vi "S8300E_Button_Test_WIH.vi"() -> ()   [LabVIEW 2011]
panel:
  out "LOG2":string
  out "Debug View":string
  in  "NG STOP":bool
  out "Pass?":bool
  out "Log":string
  out "MSG List":string[](array[string])
  out "VISA resource name out":refnum<visa-resource-name>
  out "Cmd Line":cluster{string, string, "BIST Version":string}[](array[cluster])
  out "BEGIN TIME":u32
  out "進行狀況":string
  # "Error Code:Button\nError Code:UART"
  # "2015-6-2"
  # "ShutDown Button Check"
  # "COM9 :Baud-Rate:115200"
  # "Warning:Please follow the instruction to press the Shutdown Button"
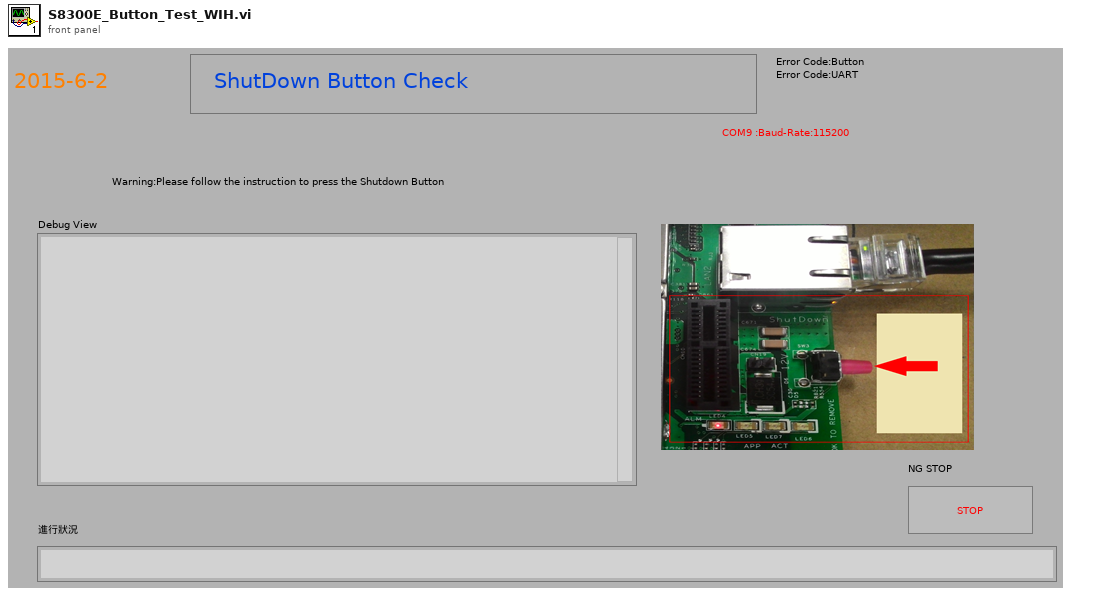
[diagram p1: front panel]
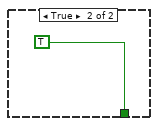
[diagram p4: hidden frame]
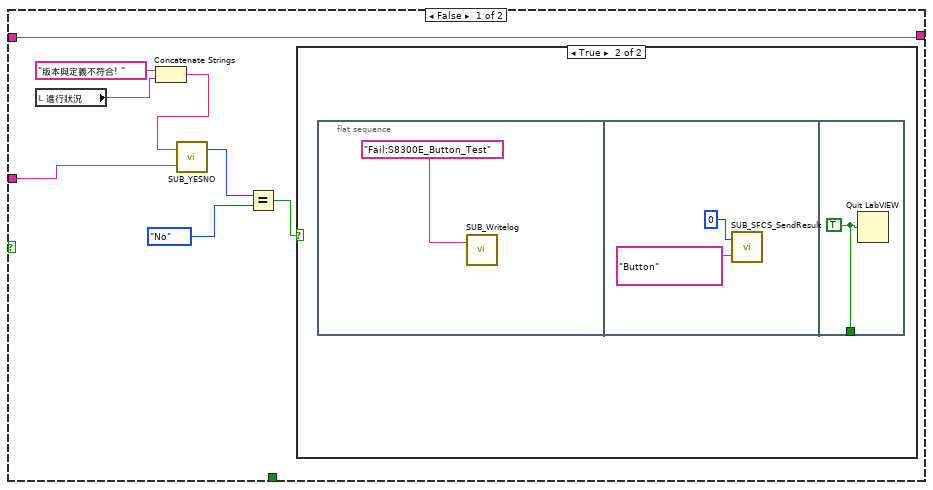
[diagram p5: hidden frame]
diagram:
  n1 = flat-sequence {
    frame #0 {
      n2 = Tick Count (ms)() -> (millisecond timer value=→"BEGIN TIME":u32)
    }
    frame #1 {
      n3 = property on="進行狀況" class="Str"("Blinking"=TRUE) -> ()  [unwired: 2 in, 2 out]
      "進行狀況" <- "進入測試準備中...." ("進行狀況")
      "Debug View" <- ""
    }
    frame #2 {
      n4 = call "SUB_SearchFile_inFolder.vi"("Search Filename in Folder"="S8300E_sfcs_misc.txt") -> ("File Existing True/Flase"=w5:bool)  [unwired: 1 in]
      n5 = case shown="False" w5 {
        frame False {
          n6 = flat-sequence {
            frame #0 {
              n7 = call "Display Message to User"() -> ()  [unwired: 10 in, 2 out]
            }
            frame #1 {
              n8 = call "SUB_Writelog.vi"("Pass/Fail"="Fail:S8300E_Button_Test") -> ()  [unwired: 2 in]
            }
            frame #2 {
              n9 = Quit LabVIEW(quit? (T)=TRUE) -> ()
            }
          }
        }
        frame True {
        }
      }
    }
    frame #3 {
      n10 = Bundle("./but.sh -r  1", "PASSED=", "0x00") -> (w13:cluster{string, string, string})  [unwired: 1 in]
      n11 = Build Array(w13) -> (→"Cmd Line":cluster{string, string, string}[])
      n12 = Build Array("正在處理 Buttun 初始值") -> (→"MSG List":string[])
    }
    frame #4 {
      n13 = call "SUB_COM1_CLOSE.vi"("VISA resource name"=refnum<visa-resource-name> "COM9") -> ()  [unwired: 3 in]
    }
    frame #5 {
      w17 = "\r"
      n14 = Concatenate Strings(w17, w17, w17, w17, w17) -> (w18:string)
      n15 = call "SUB_COM9_INIT.vi"("baud rate"=u32 115200) -> ("VISA resource name out"=w22:refnum<visa-resource-name>)  [unwired: 1 in, 1 out]
      "VISA resource name out" <- w22
      n16 = call "SUB_COM1Wrt.vi"("VISA resource name"=w22, "write buffer"=w18) -> ("duplicate VISA resource name"=w19:refnum<visa-resource-name>)  [unwired: 1 in, 1 out]
      n17 = call "SUB_ContinueCom1Read.vi"("Numeric"=1200, "duplicate VISA resource name 2"=w19) -> ()  [unwired: 1 in, 3 out]
    }
    frame #6 {
      n18 = while {
        stop <- w31 stop-if-true
        w29 = "\r"
        n19 = local read "VISA resource name out"() -> (w30:refnum<visa-resource-name>)
        n20 = Concatenate Strings(w29, w29, w29) -> (w28:string)
        n21 = Tick Count (ms)() -> (millisecond timer value=w25:u32)
        n22 = call "SUB_WR_COM1_CbyCFindString_timeout.vi"("Begin time"=w25, "Find this String"="S8300E", "Timeout Seccond"=5.0, "cmd string"=w28, "duplicate VISA resource name 2"=w30) -> ("Output String"=w23:string, "Found String"=w24:bool)  [unwired: 2 out]
        n23 = case shown="False" w24 {
          tunnel: [w33 TRUE] -> w31
          tunnel: w23 -> [w32 _]
          frame False {
            n24 = call "SUB_YESNO.vi"("Debug View"=w32, "Status"="UART無正確反應!需有S8300E字串") -> ("yes/no"=w36:enum32{"No Selection", "Yes", "No", "None"})  [unwired: 1 in]
            n25 = Equal?(x=w36, y=enum32{"No Selection", "Yes", "No", "None"}."No") -> (x = y?=w34:bool)
            n26 = case shown="True" w34 {
              tunnel: [_ w38] -> w33
              frame False {
              }
              frame True {
                n27 = flat-sequence {
                  tunnel: [w42] -> w38
                  frame #0 {
                    n28 = call "SUB_Writelog.vi"("Pass/Fail"="Fail:S8300E_Button_Test") -> ()  [unwired: 2 in]
                  }
                  frame #1 {
                    n29 = call "SUB_SFCS_SendResult.vi"("ErrorCode"="UART", "PASS_Fail (1/0)"=i8 0) -> ()  [unwired: 1 out]
                  }
                  frame #2 {
                    w42 = TRUE ("quit? (T)")
                    n30 = Quit LabVIEW(quit? (T)=w42) -> ()
                  }
                }
              }
            }
          }
          frame True {
          }
        }
      }
    }
    frame #7 {
      n31 = local read "Cmd Line"() -> (w47:cluster{string, string, "BIST Version":string}[])
      n32 = Array Size(array=w47) -> (size(s)=w46:i32)
      n33 = for {
        N: w46 -> [_]
        shift-right: [w49] -> w44
        shift-left: "" -> [w48]
        i -> [w50]
        n34 = while {
          tunnel: w50 -> [w70]
          tunnel: [w65] -> w49
          tunnel: w48 -> [w64]
          stop <- w63 stop-if-true
          n35 = local read "VISA resource name out"() -> (w71:refnum<visa-resource-name>)
          n36 = local read "Cmd Line"() -> (w69:cluster{string, string, "BIST Version":string}[])
          n37 = Index Array(array=w69, index=w70) -> (element=w68:cluster{string, string, "BIST Version":string})
          n38 = Unbundle(w68) -> (w62:string, w58:string, "BIST Version"=w54:string)
          n39 = Concatenate Strings(w62, "\r") -> (w60:string)
          n40 = call "SUB_COM1Wrt.vi"("VISA resource name"=w71, "write buffer"=w60) -> ("duplicate VISA resource name"=w59:refnum<visa-resource-name>)  [unwired: 1 in, 1 out]
          n41 = Tick Count (ms)() -> (millisecond timer value=w56:u32)
          n42 = To Upper Case(1:w54) -> (0:w53:string)
          n43 = call "SUB_READ_COM1_FindString_timeout.vi"("Find this String"=w58, "Timeout Seccond"=3.0, "Begin time"=w56, "duplicate VISA resource name 2"=w59) -> ("Output String"=w55:string)  [unwired: 1 in, 2 out]
          n44 = call "SUB_FindSpecificString.vi"("Find this String"=w58, "String data"=w55) -> ("before \"; \" string"=w67:string)  [unwired: 2 in, 1 out]
          n45 = Equal?(x=w67, y=w53) -> (x = y?=w66:bool)
          n46 = local write "Debug View"(w55) -> ()
          n47 = case shown="True" w66 {
            tunnel: w55 -> [w76 w87]
            tunnel: [w79 w86] -> w65
            tunnel: w64 -> [w79 w85]
            tunnel: [_ TRUE] -> w63
            frame False {
              n48 = local read "進行狀況"() -> (w74:string)
              n49 = Concatenate Strings("版本與定義不符合! " ("string"), w74) -> (w73:string)
              n50 = call "SUB_YESNO.vi"("Debug View"=w76, "Status"=w73) -> ("yes/no"=w78:enum32{"No Selection", "Yes", "No", "None"})  [unwired: 1 in]
              n51 = Equal?(x=w78, y=enum32{"No Selection", "Yes", "No", "None"}."No") -> (x = y?=w72:bool)
              n52 = case shown="True" w72 {
                frame False {
                }
                frame True {
                  n53 = flat-sequence {
                    tunnel: [w83] -> _
                    frame #0 {
                      n54 = call "SUB_Writelog.vi"("Pass/Fail"="Fail:S8300E_Button_Test") -> ()  [unwired: 2 in]
                    }
                    frame #1 {
                      n55 = call "SUB_SFCS_SendResult.vi"("ErrorCode"="Button", "PASS_Fail (1/0)"=i8 0) -> ()  [unwired: 1 out]
                    }
                    frame #2 {
                      w83 = TRUE ("quit? (T)")
                      n56 = Quit LabVIEW(quit? (T)=w83) -> ()
                    }
                  }
                }
              }
            }
            frame True {
              n57 = Concatenate Strings(w85, w87) -> (w86:string)
            }
          }
        }
        n58 = local read "MSG List"() -> (w52:string[])
        n59 = Index Array(array=w52, index=w50) -> (element=w51:string)
        n60 = local write "進行狀況"(w51) -> ()
      }
      "Log" <- w44
    }
    frame #8 {
    }
    frame #9 {
      n61 = property on="進行狀況" class="Str"("Blinking"=TRUE) -> ()  [unwired: 2 in, 2 out]
      n62 = local write "進行狀況"("Please Press the Button 請持壓button" ("進行狀況")) -> ()
      "Pass?" <- FALSE
    }
    frame #10 {
      n63 = while {
        stop <- w94 stop-if-true
        n64 = local read "VISA resource name out"() -> (w103:refnum<visa-resource-name>)
        n65 = Wait (ms)(milliseconds to wait=u32 20) -> ()  [unwired: 1 out]
        n66 = Concatenate Strings("./but.sh -r  1", "\r") -> (w97:string)
        n67 = call "SUB_COM1Wrt.vi"("VISA resource name"=w103, "write buffer"=w97) -> ("duplicate VISA resource name"=w100:refnum<visa-resource-name>)  [unwired: 1 in, 1 out]
        n68 = call "SUB_ContinueCom1Read.vi"("Numeric"=600, "duplicate VISA resource name 2"=w100) -> ("String"=w93:string)  [unwired: 1 in, 2 out]
        n69 = local write "Debug View"(w93) -> ()
        n70 = call "SUB_FindSpecificString.vi"("Find this String"="PASSED=0x01", "String data"=w93) -> ("before \"; \" string"=→"LOG2":string, "Found"=w96:bool)  [unwired: 2 in]
        n71 = local write "Pass?"(w96) -> ()
        n72 = Or(x=w96, y="NG STOP") -> (x .or. y?=w94:bool)
      }
    }
    frame #11 {
      n73 = local read "Pass?"() -> (w104:bool)
      n74 = case shown="False" w104 {
        frame False {
          n75 = flat-sequence {
            frame #0 {
              w106 = "\n"
              n76 = local read "LOG2"() -> (w107:string)
              n77 = local read "Log"() -> (w109:string)
              n78 = Concatenate Strings("Fail:S8300E_Button_Test" ("Pass/Fail"), w106, w109, w106, w107, w106) -> (w105:string)
              n79 = call "SUB_Writelog.vi"("Pass/Fail"=w105) -> ()  [unwired: 2 in]
            }
            frame #1 {
              n80 = call "SUB_SFCS_SendResult.vi"("ErrorCode"="Button", "PASS_Fail (1/0)"=i8 0) -> ()  [unwired: 1 out]
            }
            frame #2 {
              n81 = Quit LabVIEW(quit? (T)=TRUE) -> ()
            }
          }
        }
        frame True {
        }
      }
    }
    frame #12 {
      n82 = call "SUB_COM1_CLOSE.vi"("VISA resource name"=refnum<visa-resource-name> "COM9") -> ()  [unwired: 3 in]
    }
    frame #13 {
      w116 = "***Not Good ***" ("replace string (\"\")")
      w121 = "\n"
      n83 = local read "BEGIN TIME"() -> (w126:u32)
      n84 = Tick Count (ms)() -> (millisecond timer value=w125:u32)
      n85 = call "SUB_CAL_TESTTIME.vi"("Test Item name"="S8300E_Button_Test", "Stop tick time"=w125, "Start tick time"=w126) -> ("Test Time output"=w120:string)  [unwired: 2 in]
      n86 = local read "LOG2"() -> (w122:string)
      n87 = local read "Log"() -> (w123:string)
      n88 = Concatenate Strings("Pass:S8300E_Button_Test", w121, w123, w121, w122, w121, w120) -> (w115:string)
      n89 = call "SUB_SEARCH_REPLACE_STR.vi"("replace string (\"\")"=w116, "search string"="FAILED", "input string"=w115) -> ("result string"=w118:string)  [unwired: 2 in]
      n90 = call "SUB_SEARCH_REPLACE_STR.vi"("replace string (\"\")"=w116, "search string"="FAIL", "input string"=w118) -> ("result string"=w114:string)  [unwired: 2 in]
      n91 = call "SUB_Writelog.vi"("Pass/Fail"=w114) -> ()  [unwired: 2 in]
    }
    frame #14 {
      n92 = Request Deallocation(TRUE ("flag")) -> ()
    }
    frame #15 {
      n93 = Quit LabVIEW(quit? (T)=TRUE ("stop? (T)")) -> ()
    }
  }
